vi "PopulateHeadPropertiesInConfigDict.vi"(8 "error in (no error)":errorcluster, 11 "TopLevel in":refnum<class "TopLevel.lvclass">) -> (0 "error out":errorcluster, 2 "InkType Directory":T1[](array[typedef]), 3 "TopLevel out":refnum<class "TopLevel.lvclass">)   [LabVIEW 2022 SP3, in "TopLevel.lvclass"]
uses:
  TopLevel.lvclass
  Common/Controls/DLP_MaterialToHeadMapping--Cluster.ctl
  DLP2/DataTypes/DLP2_PrinterMaterialProperties.ctl
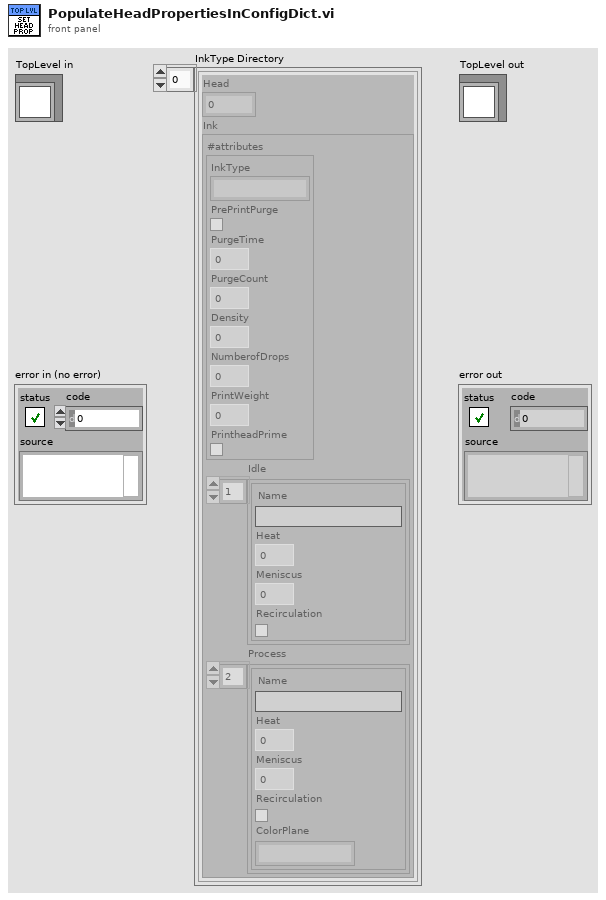
[diagram p1: front panel]
types:
  T1 = typedef "DLP_MaterialToHeadMapping--Cluster.ctl" = cluster{"Head":u8, "Ink":T2}
  T2 = typedef "DLP2_PrinterMaterialProperties.ctl" = cluster{"#attributes":cluster{"InkType":string, "PrePrintPurge":bool, "PurgeTime":dbl, "PurgeCount":i32, "Density":dbl, "NumberofDrops":i32, "PrintWeight":dbl, "PrintheadPrime":bool}, "Idle":cluster{"Name":string, "Heat":dbl, "Meniscus":dbl, "Recirculation":bool}[], "Process":cluster{"Name":string, "Heat":dbl, "Meniscus":dbl, "Recirculation":bool, "ColorPlane":string}[]}
  T3 = typedef "TD Dynamic CVT DVR--ref.ctl" = refnum<data-value>
  T4 = typedef "DLPConfig_Initialization.ctl" = cluster{"PrinterInitialization":cluster{"Printer":cluster{"#attributes":cluster{"Name":string}}, "VacPumpSet":cluster{"#attributes":cluster{"VacPumpEnable":bool, "VacPumpSpeed":dbl}}, "HIBEnable":cluster{"#attributes":cluster{"HIB1Enable":bool, "HIB2Enable":bool, "HIB3Enable":bool, "HIB4Enable":bool, "HIB5Enable":bool, "HIB6Enable":bool}}, "PrinterCompensation":T5}, "HeadSet":cluster{"HeadProperties":T6[]}, "InkSet":cluster{"Ink":T2[]}, "Troubleshooting":cluster{"PMBLogging":cluster{"#attributes":cluster{"PMBMonitorDuringPrint":bool, "PMBMonitorDuringIdle":bool, "LogSwatheInputData":bool, "LogSwatheOutputData":bool, "LogPrintheadColourPlanes":bool, "LogPMBCommunication":bool, "LogSimulatedOutput":bool, "LogAllPMBCommunicationData":bool, "LogPMBSpace":bool, "ExtendedPMBSpaceLogging":bool, "LogPMBWriteSpeed":bool, "LogUsbRetries":bool}}, "HIBLogging":cluster{"#attributes":cluster{"HIBMonitoringDuringPrint":bool, "HIBMonitoringLog":bool}}}}
  T5 = typedef "DLP2_PrinterCompensationProperties.ctl" = cluster{"#attributes":cluster{"AppName":string, "PrintWeightMultiplier":dbl, "Rotation":bool, "Driver":string, "Server":string, "Database":string, "User":string, "Password":string}}
  T6 = typedef "DLP2_PrinterHeadProperties.ctl" = cluster{"#attributes":T7}
  T7 = typedef "DLPConfig)Init_HeadPropertyAttr--Cluster.ctl" = cluster{"HeadNumber":u8, "Material":string, "HeadLocalX":dbl, "HeadLocalY":dbl, "HeadRotationAngle":dbl, "VH2L_Hi":dbl, "VH2R_Hi":dbl, "VH1LA_Hi":dbl, "VH1LB_Hi":dbl, "VH1RA_Hi":dbl, "VH1RB_Hi":dbl, "VH2L_Lo":dbl, "VH2R_Lo":dbl, "VH1LA_Lo":dbl, "VH1LB_Lo":dbl, "VH1RA_Lo":dbl, "VH1RB_Lo":dbl}
  T8 = typedef "DLPPrinterInitXML.ctl" = cluster{"PrinterInitialization":cluster{"Printer":cluster{"#attributes":cluster{"Name":string}}, "VacPumpSet":cluster{"#attributes":cluster{"VacPumpEnable":bool, "VacPumpSpeed":dbl}}, "HIBEnable":cluster{"#attributes":cluster{"HIB1Enable":bool, "HIB2Enable":bool, "HIB3Enable":bool, "HIB4Enable":bool, "HIB5Enable":bool, "HIB6Enable":bool}}, "PrinterCompensation":T5}, "HeadSet":cluster{"HeadProperties":T6[]}, "InkSet":cluster{"Ink":cluster{"#attributes":cluster{"InkType":string, "PrePrintPurge":bool, "PurgeTime":dbl, "PurgeCount":i32, "Density":dbl, "NumberofDrops":i32, "PrintWeight":dbl, "PrintheadPrime":bool}, "Idle":cluster{"Name":string, "Heat":dbl, "Meniscus":dbl, "Recirculation":bool}[], "Process":cluster{"Name":string, "Heat":dbl, "Meniscus":dbl, "Recirculation":bool, "ColorPlane":string}[]}[]}, "Troubleshooting":cluster{"PMBLogging":cluster{"#attributes":cluster{"PMBMonitorDuringPrint":bool, "PMBMonitorDuringIdle":bool, "LogSwatheInputData":bool, "LogSwatheOutputData":bool, "LogPrintheadColourPlanes":bool, "LogPMBCommunication":bool, "LogSimulatedOutput":bool, "LogAllPMBCommunicationData":bool, "LogPMBSpace":bool, "ExtendedPMBSpaceLogging":bool, "LogPMBWriteSpeed":bool, "LogUsbRetries":bool}}, "HIBLogging":cluster{"#attributes":cluster{"HIBMonitoringDuringPrint":bool, "HIBMonitoringLog":bool}}}}
  T9 = cluster{"Name":string, "Heat":dbl, "Meniscus":dbl, "Recirculation":bool}[]
  T10 = cluster{"Name":string, "Heat":dbl, "Meniscus":dbl, "Recirculation":bool, "ColorPlane":string}[]
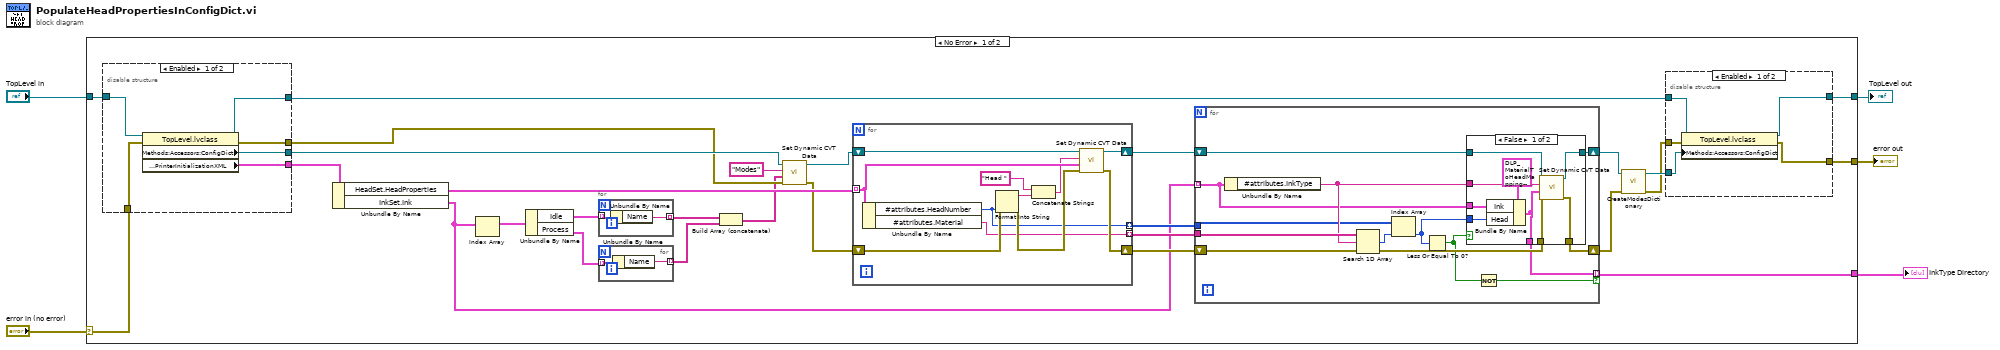
[diagram p0: block diagram]
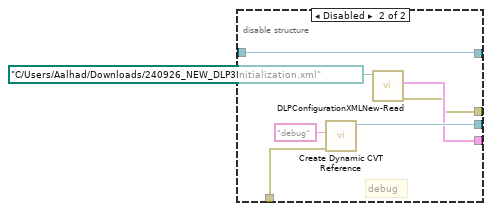
[diagram p3: hidden frame]
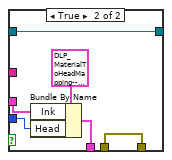
[diagram p4: hidden frame]
diagram:
  n1 = case shown="No Error" "error in (no error)" {
    selector: "error in (no error)" -> [w29 w98]
    tunnel: [w28 w98] -> w4
    tunnel: [w33 w97] -> w2
    tunnel: "TopLevel in" -> [w30 w97]
    tunnel: [w22 _] -> w1
    frame No Error {
      n2 = disable-structure shown="Enabled" {
        disable-tunnel: [w46 w53] -> w31
        disable-tunnel: w30 -> [w45 w53]
        disable-tunnel: w29 -> [w44 w50]
        disable-tunnel: [w43 w49] -> w27
        disable-tunnel: [w42 w51] -> w19
        disable-tunnel: [w41 w47] -> w18
        frame Enabled {
          n3 = property class="TopLevel.lvclass"(reference=w45, error in=w44) -> (reference out=w46:refnum<class "TopLevel.lvclass">, error out=w41:errorcluster, "Methods:Accessors:ConfigDict"=w42:T3, "Methods:Accessors:PrinterInitializationXML"=w43:T4)
        }
        frame Disabled {
          # "debug"
          n4 = call <vilib>:"Create Dynamic CVT Reference.vi"("error in (no error)"=w50, "DictName"="debug") -> ("dCVT DVR out"=w51:T3)  [unwired: 8 in, 1 out]
          n5 = call "DLPConfigurationXMLNew-Read.vi"("XML File Path"=path "C:/Users/Aalhad/Downloads/240926_NEW_DLP3Initialization.xml") -> ("error out"=w47:errorcluster, "data"=w49:T8)  [unwired: 8 in, 1 out]
        }
      }
      n6 = Unbundle By Name(w27) -> ("HeadSet.HeadProperties"=w32:T6[], "InkSet.Ink"=w21:T2[])
      n7 = Index Array(array=w21) -> (element=w20:T2)  [unwired: 1 in]
      n8 = Unbundle By Name(w20) -> ("Idle"=w13:T9, "Process"=w17:T10)
      n9 = for {
        tunnel: w13 -> [w55] mode=indexing
        tunnel: [w54] -> w12 mode=indexing
        n10 = Unbundle By Name(w55) -> ("Name"=w54:string)
      }
      n11 = for {
        tunnel: w17 -> [w57] mode=indexing
        tunnel: [w56] -> w11 mode=indexing
        n12 = Unbundle By Name(w57) -> ("Name"=w56:string)
      }
      n13 = Build Array (concatenate)(w12, w11) -> (w10:string[])
      n14 = call <vilib>:"Set Dynamic CVT Data.vi"("error in (no error)"=w18, "value"=w10, "DataName"="Modes", "dCVT DVR"=w19) -> ("error out"=w16:errorcluster, "dCVT DVR out"=w15:T3)  [unwired: 5 in, 1 out]
      n15 = for {
        tunnel: w32 -> [w93] mode=indexing
        shift-right: [w95] -> w26
        shift-left: w15 -> [w96]
        shift-right: [w94] -> w25
        shift-left: w16 -> [w88]
        tunnel: [w87] -> w24 mode=indexing
        tunnel: [w86] -> w23 mode=indexing
        n16 = Unbundle By Name(w93) -> ("#attributes.HeadNumber"=w87:u8, "#attributes.Material"=w86:string)
        n17 = Format Into String(error in=w88, w87) -> (resulting string=w91:string, error out=w89:errorcluster)  [unwired: 2 in]
        n18 = Concatenate Strings("Head " ("string"), w91) -> (w90:string)
        n19 = call <vilib>:"Set Dynamic CVT Data.vi"("error in (no error)"=w89, "value"=w93, "DataName"=w90, "dCVT DVR"=w96) -> ("error out"=w94:errorcluster, "dCVT DVR out"=w95:T3)  [unwired: 5 in, 1 out]
      }
      n20 = for {
        shift-right: [w69] -> w9
        shift-left: w26 -> [w70]
        shift-right: [w67] -> w7
        shift-left: w25 -> [w68]
        tunnel: w21 -> [w62] mode=indexing
        tunnel: w24 -> [w63]
        tunnel: w23 -> [w66]
        tunnel: [w61] -> w22 mode=indexing if=w58
        n21 = Unbundle By Name(w62) -> ("#attributes.InkType"=w65:string)
        n22 = Search 1D Array(1D array=w66, element=w65) -> (index of element=w64:i32)  [unwired: 1 in]
        n23 = Index Array(array=w63, index=w64) -> (element=w60:u8)
        n24 = Less Or Equal To 0?(x=w60) -> (x <= 0?=w59:bool)
        n25 = case shown="False" w59 {
          tunnel: w70 -> [w79 w85]
          tunnel: [w78 w85] -> w69
          tunnel: w68 -> [w77 w84]
          tunnel: [w76 w84] -> w67
          tunnel: w65 -> [w75 _]
          tunnel: w62 -> [w73 w82]
          tunnel: [w72 w80] -> w61
          tunnel: w60 -> [w71 w81]
          frame False {
            n26 = Bundle By Name(cluster=T1 {"Head"=0, "Ink"={"#attributes"={"InkType"="", "PrePrintPurge"=FALSE, "PurgeTime"=0.0, "PurgeCount"=0, "Density"=0.0, "NumberofDrops"=0, "PrintWeight"=0.0, "PrintheadPrime"=FALSE}, "Idle"=[], "Process"=[]}}, "Ink"=w73, "Head"=w71) -> (w72:T1)
            n27 = call <vilib>:"Set Dynamic CVT Data.vi"("error in (no error)"=w77, "value"=w72, "DataName"=w75, "dCVT DVR"=w79) -> ("error out"=w76:errorcluster, "dCVT DVR out"=w78:T3)  [unwired: 5 in, 1 out]
          }
          frame True {
            n28 = Bundle By Name(cluster=T1 {"Head"=0, "Ink"={"#attributes"={"InkType"="", "PrePrintPurge"=FALSE, "PurgeTime"=0.0, "PurgeCount"=0, "Density"=0.0, "NumberofDrops"=0, "PrintWeight"=0.0, "PrintheadPrime"=FALSE}, "Idle"=[], "Process"=[]}}, "Ink"=w82, "Head"=w81) -> (w80:T1)
          }
        }
        n29 = Not(x=w59) -> (.not. x?=w58:bool)
      }
      n30 = call "CreateModesDictionary.vi"("error in (no error)"=w7, "Data Value Reference in"=w9) -> ("error out"=w6:errorcluster, "Data Value Reference out"=w8:T3)  [unwired: 8 in]
      n31 = disable-structure shown="Enabled" {
        disable-tunnel: [w38 w40] -> w33
        disable-tunnel: w31 -> [w37 w40]
        disable-tunnel: [w36 w39] -> w28
        disable-tunnel: w8 -> [w35 _]
        disable-tunnel: w6 -> [w34 w39]
        frame Enabled {
          n32 = property class="TopLevel.lvclass"(reference=w37, error in=w34, "Methods:Accessors:ConfigDict"=w35) -> (reference out=w38:refnum<class "TopLevel.lvclass">, error out=w36:errorcluster)
        }
        frame Disabled {
          # "debug"
        }
      }
    }
    frame Error {
    }
  }
  "error out" <- w4
  "TopLevel out" <- w2
  "InkType Directory" <- w1
